vi "user process.vi"(8 "error in":errorcluster, 10 "Parameters to process":T2, 11 "Custom Temperature Controller runtime in":refnum<class "Custom Temperature Controller runtime.lvclass">) -> (0 "error out":errorcluster, 2 "Results from processing":T1, 3 "Custom Temperature Controller runtime out":refnum<class "Custom Temperature Controller runtime.lvclass">)   [LabVIEW 2015, in "Custom Temperature Controller runtime.lvclass"]
uses:
  Custom Temperature Controller runtime.lvclass
  parameter user data.ctl
  result user data.ctl
  <vilib>/addons/control/pid/pid.llb/PID (DBL).vi
  <vilib>/addons/control/pid/NI_PID_pid.lvlib
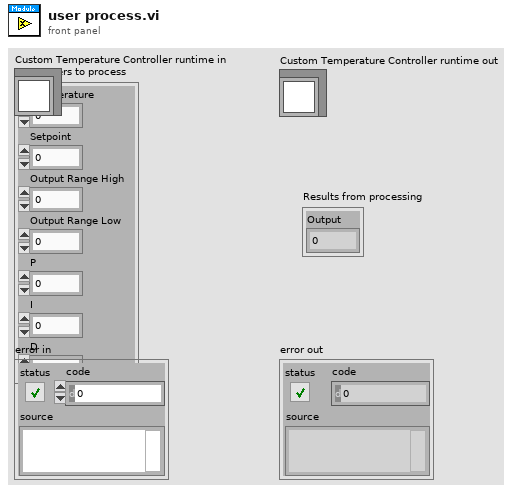
[diagram p1: front panel]
types:
  T1 = typedef "Custom Temperature Controller runtime.lvclass/result user data.ctl" = cluster{"Output":dbl}
  T2 = typedef "Custom Temperature Controller runtime.lvclass/parameter user data.ctl" = cluster{"Temperature":dbl, "Setpoint":dbl, "Output Range High":dbl, "Output Range Low":dbl, "P":dbl, "I":dbl, "D":dbl}
  T3 = cluster{"proportional gain (Kc)":dbl, "integral time (Ti, min)":dbl, "derivative time (Td, min)":dbl}
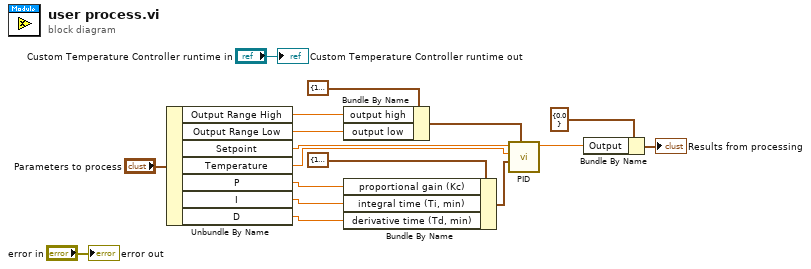
[diagram p0: block diagram]
diagram:
  n1 = Unbundle By Name("Parameters to process") -> ("Output Range High"=w5:dbl, "Output Range Low"=w4:dbl, "Setpoint"=w12:dbl, "Temperature"=w11:dbl, "P"=w3:dbl, "I"=w2:dbl, "D"=w1:dbl)
  n2 = Bundle By Name(cluster=cluster{"output high":dbl, "output low":dbl} {"output high"=100.0, "output low"=-100.0} ("output range"), "output high"=w5, "output low"=w4) -> (w6:cluster{"output high":dbl, "output low":dbl})
  n3 = Bundle By Name(cluster=T3 {"proportional gain (Kc)"=1.0, "integral time (Ti, min)"=0.01, "derivative time (Td, min)"=0.0} ("PID gains"), "proportional gain (Kc)"=w3, "integral time (Ti, min)"=w2, "derivative time (Td, min)"=w1) -> (w8:T3)
  n4 = call-poly <vilib>:"PID.vi"("output range"=w6, "PID gains"=w8, "process variable"=w11, "setpoint"=w12) -> ("output"=w10:dbl)  [unwired: 6 in, 1 out]
  n5 = Bundle By Name(cluster=T1 {"Output"=0.0} ("Results from processing"), "Output"=w10) -> (→"Results from processing":T1)
  "error out" <- "error in"
  "Custom Temperature Controller runtime out" <- "Custom Temperature Controller runtime in"
